vi "__uintGCD.vi"(8 "Base (decimal)":T1=10 items=["Binary"=2, "Octal"=8, "Decimal"=10, "Hexadecimal"=16, "Hexatrigesimal"=36, "ASCII"=64], 10 "Uint2 in":u8[](array[numeric])=[0], 11 "Uint1 in":u8[](array[numeric])=[0]) -> (0 "Timing":u32, 3 "GCD(Int1,Int2)":u8[](array[numeric]))   [LabVIEW 2011, in "UintClass.lvclass"]
uses:
  UintClass.lvclass
  enumBase.ctl
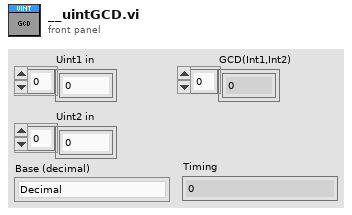
[diagram p1: front panel]
types:
  T1 = typedef "UintClass.lvclass/enumBase.ctl" = u16
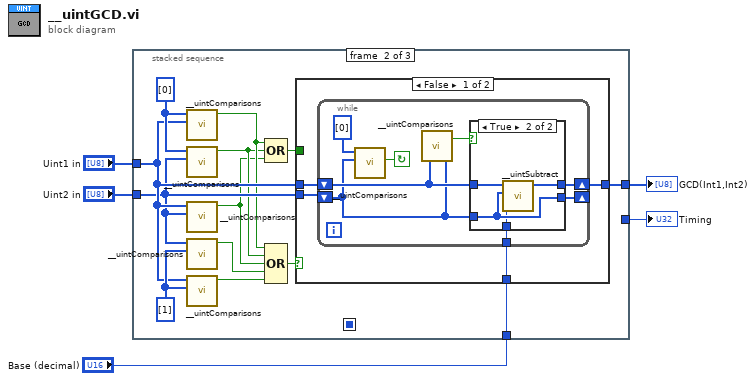
[diagram p0: block diagram]
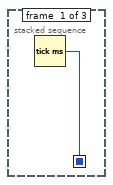
[diagram p2: hidden frame]
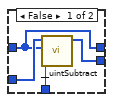
[diagram p3: hidden frame]
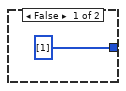
[diagram p5: hidden frame]
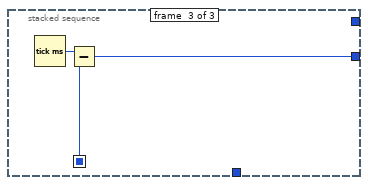
[diagram p6: hidden frame]
diagram:
  n1 = stacked-sequence {
    seq-local: [w6 _ _] -> [_ _ w46]
    tunnel: "Uint1 in" -> [_ w16 _]
    tunnel: "Uint2 in" -> [_ w15 _]
    tunnel: [_ w14 _] -> w3
    tunnel: "Base (decimal)" -> [_ w7 _]
    tunnel: [_ _ w45] -> w1
    frame #0 {
      n2 = Tick Count (ms)() -> (millisecond timer value=w6:u32)
    }
    frame #1 {
      w18 = u8[] [1] ("Uint2 in")
      w19 = u8[] [0] ("Uint2 in")
      n3 = call "__uintComparisons.vi"("Uint2 in"=w16, "Uint1 in"=w19) -> ("Uint1 = Uint2"=w11:bool)  [unwired: 3 in, 6 out]
      n4 = call "__uintComparisons.vi"("Uint2 in"=w15, "Uint1 in"=w19) -> ("Uint1 = Uint2"=w10:bool)  [unwired: 3 in, 6 out]
      n5 = call "__uintComparisons.vi"("Uint2 in"=w15, "Uint1 in"=w16) -> ("Uint1 = Uint2"=w9:bool)  [unwired: 3 in, 6 out]
      n6 = call "__uintComparisons.vi"("Uint2 in"=w18, "Uint1 in"=w15) -> ("Uint1 = Uint2"=w12:bool)  [unwired: 3 in, 6 out]
      n7 = call "__uintComparisons.vi"("Uint2 in"=w18, "Uint1 in"=w16) -> ("Uint1 = Uint2"=w13:bool)  [unwired: 3 in, 6 out]
      n8 = Compound Arithmetic op=OR(w11, w10, w9) -> (w8:bool)
      n9 = Compound Arithmetic op=OR(w11, w10, w9, w12, w13) -> (w17:bool)
      n10 = case shown="False" w17 {
        tunnel: w16 -> [w23 w41]
        tunnel: w15 -> [w22 _]
        tunnel: [w21 w42] -> w14
        tunnel: w8 -> [_ w40]
        tunnel: w7 -> [w20 _]
        frame False {
          n11 = while {
            shift-right: [w29] -> w21
            shift-left: w23 -> [w25]
            shift-right: [w28] -> _
            shift-left: w22 -> [w24]
            tunnel: w20 -> [w27]
            stop <- w31 continue-if-true
            n12 = call "__uintComparisons.vi"("Uint2 in"=w24, "Uint1 in"=u8[] [0] ("Uint2 in")) -> ("Uint1 != Uint2"=w31:bool)  [unwired: 3 in, 6 out]
            n13 = call "__uintComparisons.vi"("Uint2 in"=w24, "Uint1 in"=w25) -> ("Uint1 > Uint2"=w26:bool)  [unwired: 3 in, 6 out]
            n14 = case shown="True" w26 {
              tunnel: w24 -> [w35 w37]
              tunnel: w25 -> [w33 w39]
              tunnel: [w33 w38] -> w29
              tunnel: [w34 w37] -> w28
              tunnel: w27 -> [w32 w36]
              frame False {
                n15 = call "__uintSubtract.vi"("Base (decimal)"=w32, "Uint2 in"=w33, "Uint1 in"=w35) -> ("Uint1 - Uint2"=w34:u8[])  [unwired: 7 in, 1 out]
              }
              frame True {
                n16 = call "__uintSubtract.vi"("Base (decimal)"=w36, "Uint2 in"=w37, "Uint1 in"=w39) -> ("Uint1 - Uint2"=w38:u8[])  [unwired: 7 in, 1 out]
              }
            }
          }
        }
        frame True {
          n17 = case shown="True" w40 {
            tunnel: [u8[] [1] ("Uint1 in") w44] -> w42
            tunnel: w41 -> [_ w44]
            frame False {
            }
            frame True {
            }
          }
        }
      }
    }
    frame #2 {
      n18 = Tick Count (ms)() -> (millisecond timer value=w47:u32)
      n19 = Subtract(x=w47, y=w46) -> (x-y=w45:u32)
    }
  }
  "GCD(Int1,Int2)" <- w3
  "Timing" <- w1
